vi "SPI Number.vi"(4 "SPI in":refnum<class "SPI.lvclass">) -> (7 "SPI #":T1=-1)   [LabVIEW 2020, in "CTI.lvlib" / "SPI.lvclass"]
uses:
  SPI.lvclass
  SPI Number.ctl
  SPI.lvclass/SPI.ctl
  CTI.lvlib
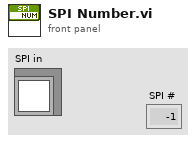
[diagram p1: front panel]
types:
  T1 = typedef "CTI.lvlib/SPI Number.ctl" = i8
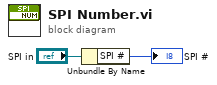
[diagram p0: block diagram]
diagram:
  n1 = Unbundle By Name("SPI in") -> ("SPI #"=→"SPI #":T1)
